vi "Read Monitor notifier.vi"(0 "HGF_DSCMonitor.lvclass in":refnum<class "HGF_DSCMonitor.lvclass">, 5 "error in (no error)":errorcluster) -> (14 "HGF_DSCMonitor.lvclass out":refnum<class "HGF_DSCMonitor.lvclass">, 17 "Monitor Queue":refnum<queue>, 19 "error out":errorcluster)   [LabVIEW 2009]
uses:
  HGF_DSCMonitor.lvclass
  HGF_BaseClasses/HGF_NetworkVisitor/HGF_NetworkVisitor.lvclass
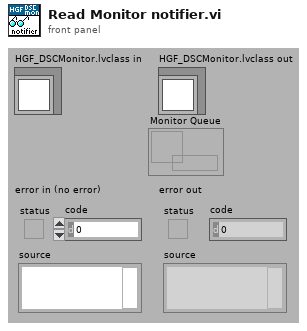
[diagram p1: front panel]
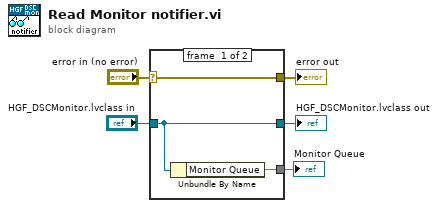
[diagram p0: block diagram]
diagram:
  n1 = case shown="No Error" "error in (no error)" {
    selector: "error in (no error)" -> [w8 w9]
    tunnel: [w8 w9] -> w4
    tunnel: [w7 w10] -> w2
    tunnel: "HGF_DSCMonitor.lvclass in" -> [w7 w10]
    tunnel: [w6 _] -> w1
    frame #0 {
      n2 = Unbundle By Name(w7) -> ("Monitor Queue"=w6)
    }
    frame #1 {
    }
  }
  "error out" <- w4
  "HGF_DSCMonitor.lvclass out" <- w2
  "Monitor Queue" <- w1
